vi "Waveform Generation Using Formula.vi"() -> ()   [LabVIEW 2020]
doc: "Demonstrates the use of the Formula Waveform VI and shows the use of many predefined variables used within the formula string of the Formula Waveform VI."
uses:
  <vilib>/measure/NI_MAPro.lvlib
panel:
  in  "Formula":string(combo)="a*sin(w*t)*(3-sin(10*pi(1)*t))"
  out "Waveform Graph":waveform(dbl)(graph)
  # "Overview: Demonstrates the use of the Formula Waveform VI.\nRequirements: LabVIEW Full Development System\nInstructions:\n1. Select a Formula value and run the VI.\n2. Note that if you select the 'invalid formula', the VI generates an error."
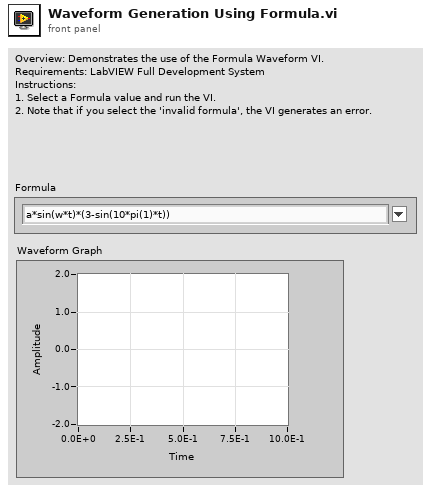
[diagram p1: front panel]
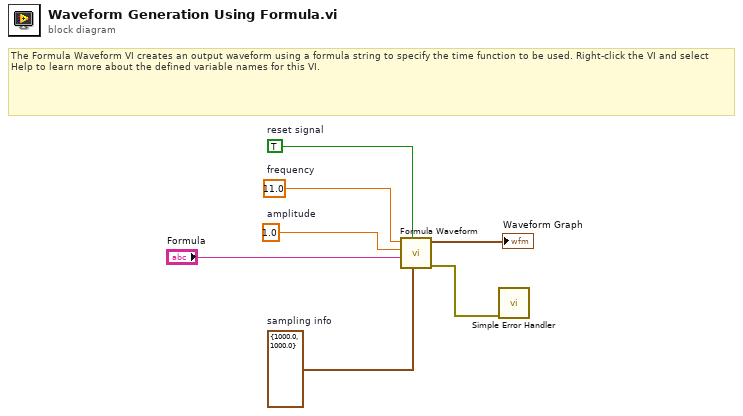
[diagram p0: block diagram]
diagram:
  w4 = 1.0  # amplitude
  w3 = TRUE  # reset signal
  w5 = 11.0  # frequency
  w6 = cluster{"Fs":dbl, "#s":dbl} {"Fs"=1000.0, "#s"=1000.0}  # sampling info
  # "The Formula Waveform VI creates an output waveform using a formula string to specify the time function to be used. Right-click the VI and select Help to learn more about the defined variable names for this VI."
  n1 = call <vilib>:"Formula Waveform.vi"("sampling info"=w6, "reset signal"=w3, "formula"="Formula", "amplitude"=w4, "frequency"=w5) -> ("error out"=w2:errorcluster, "signal out"=→"Waveform Graph":waveform(dbl))  [unwired: 5 in]
  n2 = call <vilib>:"Simple Error Handler.vi"("error in (no error)"=w2) -> ()  [unwired: 4 in, 5 out]
